vi "FindHome.vi"(0 "axis in":cluster{"keyHandle":u32, "nodeId":u16}={"keyHandle"=0, "nodeId"=1}, 5 "homingParameter":T1, 7 "homing Method":i8(ring) items=["No homing operation required"=0, "Negative Limit Switch & Index"=1, "Positive Limit Switch & Index"=2, "Home Switch Positive Speed & Index"=7, "Home Switch Negative Speed & Index"=11, "Negative Limit Switch"=17, "Positive Limit Switch"=18, "Home Switch Positive Speed"=23, "Home Switch Negative Speed"=27, "Index Negative Speed"=33, "Index Positive Speed"=34, "Actual Position"=35, "Current Threshold Positive Speed & Index"=-1, "Current Threshold Negative Speed & Index"=-2, "Current Threshold Positive Speed"=-3, "Current Threshold Negative Speed"=-4], 9 "timeout":u32, 11 "error in (no error)":errorcluster) -> (4 "axis out":cluster{"keyHandle":u32, "nodeId":u16}={"keyHandle"=0, "nodeId"=1}, 15 "error out":errorcluster)   [LabVIEW 2019, in "maxonEPOS.lvlib"]
doc: "<B>FindHome</B> searchs the home position with the defined homing method. Before the movement starts, the homing parameter are written."
uses:
  Examples/maxonEPOS.lvlib
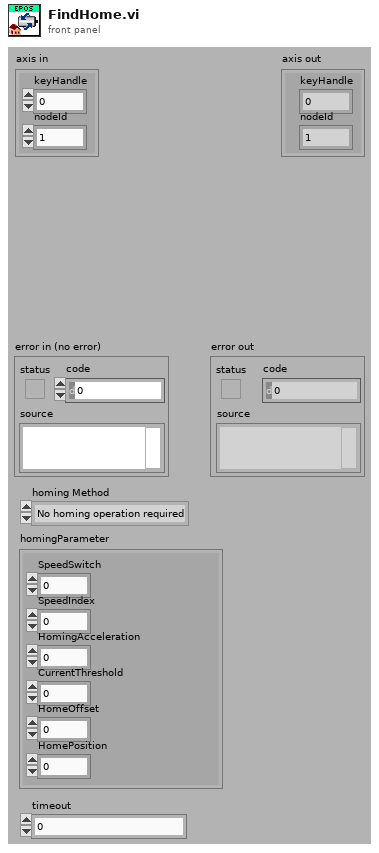
[diagram p1: front panel]
types:
  T1 = cluster{"SpeedSwitch":u32, "SpeedIndex":u32, "HomingAcceleration":u32, "CurrentThreshold":u16, "HomeOffset":i32, "HomePosition":i32}
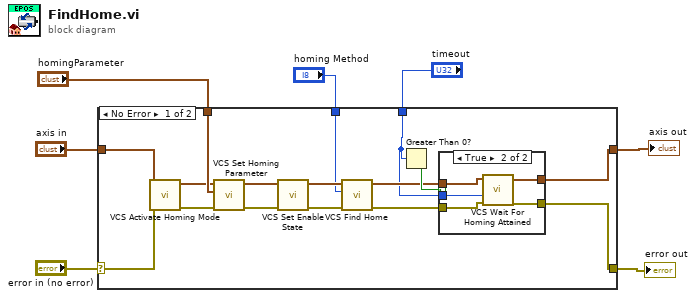
[diagram p0: block diagram]
diagram:
  n1 = case shown="No Error" "error in (no error)" {
    selector: "error in (no error)" -> [w14 w32]
    tunnel: [w8 w32] -> w6
    tunnel: [w9 w31] -> w5
    tunnel: "axis in" -> [w15 w31]
    tunnel: "homingParameter" -> [w19 _]
    tunnel: "homing Method" -> [w18 _]
    tunnel: "timeout" -> [w10 _]
    frame No Error {
      n2 = call "VCS Activate Homing Mode.vi"("error in (no error)"=w14, "axis in"=w15) -> ("error out"=w17:errorcluster, "axis out"=w16:cluster{"keyHandle":u32, "nodeId":u16})  [unwired: 8 in]
      n3 = call "VCS Set Homing Parameter.vi"("error in (no error)"=w17, "homingParameter"=w19, "axis in"=w16) -> ("error out"=w23:errorcluster, "axis out"=w22:cluster{"keyHandle":u32, "nodeId":u16})  [unwired: 7 in]
      n4 = call "VCS Set Enable State.vi"("error in (no error)"=w23, "axis in"=w22) -> ("error out"=w21:errorcluster, "axis out"=w20:cluster{"keyHandle":u32, "nodeId":u16})  [unwired: 8 in]
      n5 = call "VCS Find Home.vi"("error in (no error)"=w21, "homing Method"=w18, "axis in"=w20) -> ("error out"=w12:errorcluster, "axis out"=w11:cluster{"keyHandle":u32, "nodeId":u16})  [unwired: 7 in]
      n6 = Greater Than 0?(x=w10) -> (x > 0?=w13:bool)
      n7 = case shown="True" w13 {
        tunnel: [w24 w30] -> w9
        tunnel: [w25 w29] -> w8
        tunnel: w12 -> [w25 w28]
        tunnel: w11 -> [w24 w26]
        tunnel: w10 -> [_ w27]
        frame False {
        }
        frame True {
          n8 = call "VCS Wait For Homing Attained.vi"("error in (no error)"=w28, "timeout"=w27, "axis in"=w26) -> ("error out"=w29:errorcluster, "axis out"=w30:cluster{"keyHandle":u32, "nodeId":u16})  [unwired: 7 in]
        }
      }
    }
    frame Error {
    }
  }
  "error out" <- w6
  "axis out" <- w5
